vi "OAT Polar Set Rotating Direction.vi"(9 "shaft rotating direction":u16(ring) items=["CCW", "CW"], 11 "probe position":u16) -> (1 "select type":i32, 2 "label out":string[](array[string]), 3 "label justification":T1(array[cluster]))   [LabVIEW 2017]
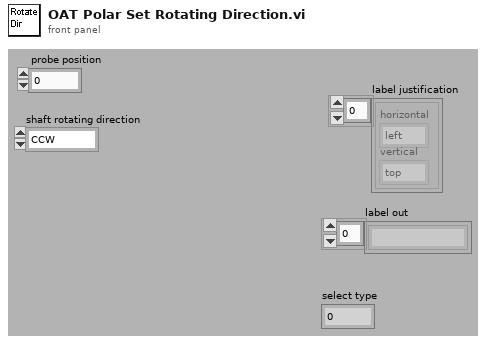
[diagram p1: front panel]
types:
  T1 = cluster{"horizontal":enum16{"left", "center", "right"}, "vertical":enum16{"top", "center", "bottom"}}[]
  T2 = cluster{"horizontal":enum16{"left", "center", "right"}, "vertical":enum16{"top", "center", "bottom"}}[][]
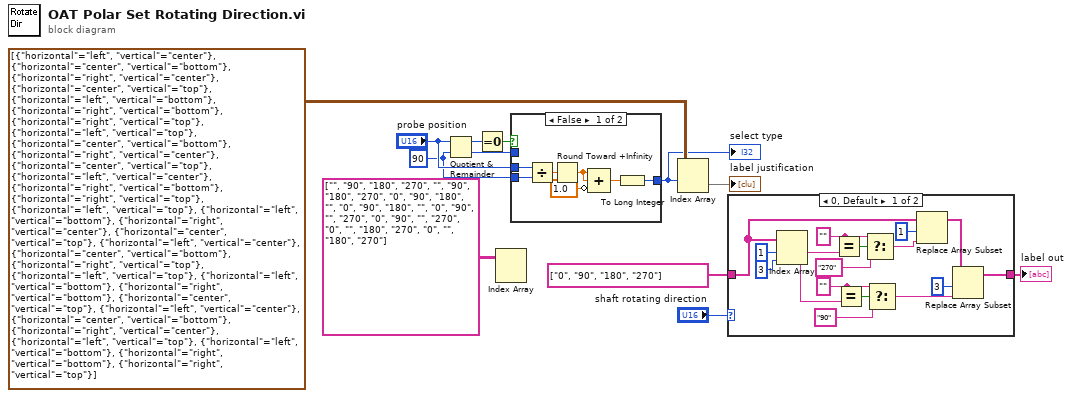
[diagram p0: block diagram]
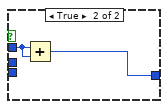
[diagram p2: hidden frame]
diagram:
  w6 = u16 90 ("y")
  n1 = Quotient & Remainder(x="probe position", y=w6) -> (x-y*floor(x/y)=w10:u16, floor(x/y)=w8:u16)
  n2 = Equal To 0?(x=w10) -> (x = 0?=w9:bool)
  n3 = Index Array(array=string[][] [["", "90", "180", "270"], ["", "90", "180", "270"], ["0", "90", "180", ""], ["0", "90", "180", ""], ["0", "90", "", "270"], ["0", "90", "", "270"], ["0", "", "180", "270"], ["0", "", "180", "270"]] ("axis labels")) -> ()  [unwired: 2 in, 1 out]
  n4 = case shown="False" w9 {
    tunnel: w8 -> [_ w21]
    tunnel: [w13 w20] -> w2
    tunnel: "probe position" -> [w19 _]
    tunnel: w6 -> [w18 _]
    frame False {
      n5 = Divide(x=w19, y=w18) -> (x/y=w17:dbl)
      n6 = Round Toward +Infinity(x=w17) -> (ceil(x): smallest int >= x=w16:dbl)
      n7 = Compound Arithmetic op=ADD(w16, w16, invert 1.0 ("value")) -> (w14:dbl)
      n8 = To Long Integer(number=w14) -> (32bit integer=w13:i32)
    }
    frame True {
      n9 = Add(x=w21, y=w21) -> (x+y=w20:u16)
    }
  }
  "select type" <- w2
  n10 = Index Array(array=T2 [[{"horizontal"=enum."left", "vertical"=enum."center"}, {"horizontal"=enum."center", "vertical"=enum."bottom"}, {"horizontal"=enum."right", "vertical"=enum."center"}, {"horizontal"=enum."center", "vertical"=enum."top"}], [{"horizontal"=enum."left", "vertical"=enum."bottom"}, {"horizontal"=enum."right", "vertical"=enum."bottom"}, {"horizontal"=enum."right", "vertical"=enum."top"}, {"horizontal"=enum."left", "vertical"=enum."top"}], [{"horizontal"=enum."center", "vertical"=enum."bottom"}, {"horizontal"=enum."right", "vertical"=enum."center"}, {"horizontal"=enum."center", "vertical"=enum."top"}, {"horizontal"=enum."left", "vertical"=enum."center"}], [{"horizontal"=enum."right", "vertical"=enum."bottom"}, {"horizontal"=enum."right", "vertical"=enum."top"}, {"horizontal"=enum."left", "vertical"=enum."top"}, {"horizontal"=enum."left", "vertical"=enum."bottom"}], [{"horizontal"=enum."right", "vertical"=enum."center"}, {"horizontal"=enum."center", "vertical"=enum."top"}, {"horizontal"=enum."left", "vertical"=enum."center"}, {"horizontal"=enum."center", "vertical"=enum."bottom"}], [{"horizontal"=enum."right", "vertical"=enum."top"}, {"horizontal"=enum."left", "vertical"=enum."top"}, {"horizontal"=enum."left", "vertical"=enum."bottom"}, {"horizontal"=enum."right", "vertical"=enum."bottom"}], [{"horizontal"=enum."center", "vertical"=enum."top"}, {"horizontal"=enum."left", "vertical"=enum."center"}, {"horizontal"=enum."center", "vertical"=enum."bottom"}, {"horizontal"=enum."right", "vertical"=enum."center"}], [{"horizontal"=enum."left", "vertical"=enum."top"}, {"horizontal"=enum."left", "vertical"=enum."bottom"}, {"horizontal"=enum."right", "vertical"=enum."bottom"}, {"horizontal"=enum."right", "vertical"=enum."top"}]] ("label justification"), index (row)=w2) -> (element=→"label justification":T1)  [unwired: 1 in]
  n11 = case shown="0, Default" "shaft rotating direction" {
    tunnel: string[] ["0", "90", "180", "270"] -> [w33 w39]
    tunnel: [w22 w39] -> w11
    frame 0, Default {
      w30 = "" ("y")
      w34 = "" ("y")
      n12 = Index Array(array=w33, index #1=1 ("index"), index #2=3 ("index")) -> (element #1=w35:string, element #2=w26:string)
      n13 = Equal?(x=w34, y=w35) -> (x = y?=w36:bool)
      n14 = Equal?(x=w30, y=w26) -> (x = y?=w27:bool)
      n15 = Select(t=w34, s=w36, f="270") -> (s? t:f=w31:string)
      n16 = Select(t=w30, s=w27, f="90") -> (s? t:f=w23:string)
      n17 = Replace Array Subset(array=w33, new element=w31, index=1) -> (w25:string[])
      n18 = Replace Array Subset(array=w25, new element=w23, index=3) -> (w22:string[])
    }
    frame 1 {
    }
  }
  "label out" <- w11
